vi "PID Sample Test.vi"(8 "error in":errorcluster, 11 "classes in":T3) -> (0 "error out":errorcluster, 3 "classes out":T3)   [LabVIEW 2011]
uses:
  Controls/Class Objects.ctl
  Modules/File/Configuration/Configuration.lvclass
  Modules/Hardware/Power Supply/Power Supply.lvclass
  Modules/Hardware/Mass Flow Controller/Mass Flow Controller.lvclass
  Modules/Hardware/Valve Controller/Valve Controller.lvclass
  Modules/Hardware/Multimeter/Multimeter.lvclass
  Modules/Hardware/Vapour Generator/Vapour Generator.lvclass
  Modules/File/TDMS/TDMS.lvclass
  Modules/Hardware/PID/PID.lvclass
  Modules/Hardware/Owlstone GEN-SYS/Gen-Sys Setpoints.ctl
  Modules/Hardware/Vapour Generator/Gas Output.ctl
  Modules/Hardware/Owlstone GEN-SYS/Owlstone GEN-SYS.lvclass
  Functional Global Data/Device Params Global.ctl
  Controls/TDMS File Handling.ctl
panel:
  out "Gas Output":T1 {"Relative Humidity (%)" format="%#.4g"; "Flow Rate (ml/min)" format="%#.0f"; "Concentration (ppm)" format="%#.2g"}
  in  "Owlstone-GEN-SYS Setpoints":T2={"OVG-4"={"Oven Temperature"=25, "Sample Flow Rate"=50, "Split Flow Status"=0, "Split Flow Rate"=300}, "OHG-4"={"Wet Air Flow"=300}} {"OHG-4"."Wet Air Flow" min=300 max=3000 scale=300.0..3000.0; "OVG-4"."Split Flow Status" items=["Closed", "Open"]; "OVG-4"."Split Flow Rate" min=300 max=3000 scale=300.0..3000.0; "OVG-4"."Sample Flow Rate" min=50 max=500 scale=50.0..500.0; "OVG-4"."Oven Temperature" min=25 max=100 scale=25.0..100.0}
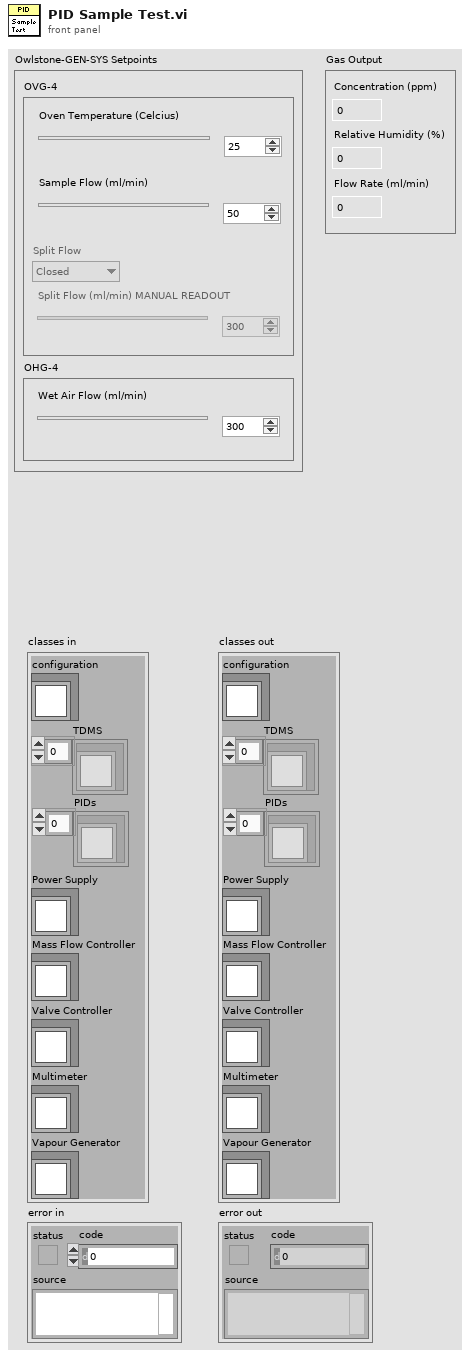
[diagram p1: front panel]
types:
  T1 = typedef "Vapour Generator.lvclass/Gas Output.ctl" = cluster{"Concentration (ppm)":dbl, "Flow Rate (ml/min)":dbl, "Relative Humidity (%)":dbl}
  T2 = typedef "Owlstone GEN-SYS.lvclass/Gen-Sys Setpoints.ctl" = cluster{"OVG-4":cluster{"Oven Temperature":i32, "Sample Flow Rate":i32, "Split Flow Status":u16, "Split Flow Rate":i32}, "OHG-4":cluster{"Wet Air Flow":i32}}
  T3 = typedef "Class Objects.ctl" = cluster{"configuration":refnum<class "Configuration.lvclass">, "TDMS":refnum<class "TDMS.lvclass">[], "Power Supply":refnum<class "Power Supply.lvclass">, "Mass Flow Controller":refnum<class "Mass Flow Controller.lvclass">, "Valve Controller":refnum<class "Valve Controller.lvclass">, "Multimeter":refnum<class "Multimeter.lvclass">, "Vapour Generator":refnum<class "Vapour Generator.lvclass">, "PIDs":refnum<class "PID.lvclass">[]}
  T4 = typedef "Device Params Global.ctl" = enum16{"Initialize", "Get Device Settings", "Get Device Connections", "Set Device Settings", "Set Device Connections", "Get All Device Properties"}
  T5 = typedef "TDMS File Handling.ctl" = enum16{"Add TDMS File", "Get Active TDMS File", "Set Active TDMS File", "Set Active TDMS File Index"}
  T6 = typedef "Device Settings.ctl" = cluster{"PID":cluster{"B-M PID":T7, "INL PID":T8}, "Power Supply":cluster{"Source Value":dbl, "Source Value Units":T9, "Source Mode":T10, "Limits":T11, "Output":bool}, "Mass Flow Controller":cluster{"MFC Flow Rate":dbl, "MFC Valve Status":T14}, "Valve Controller":cluster{"Valve Assembly":T15}, "Multimeter":cluster{"Agilent 3458A":cluster{"Measurement Configuration":T17, "Measurement Integration":T18}}, "Vapour Generator":cluster{"Owlstone Permeation Tube":T19, "Owlstone GEN-SYS Setpoints":T2}}
  T7 = typedef "Baseline Mocon piD-Tech plus.lvclass/Settings.ctl" = cluster{"Detector Sampling Frequency":dbl}
  T8 = typedef "INL PID.lvclass/Settings.ctl" = cluster{"Sampling Frequency":dbl, "Integration Time":dbl, "Integration Periods":u8, "Grid Voltage":dbl}
  T9 = typedef "Power Supply.lvclass/Source Units.ctl" = enum16{"volts", "millivolts", "microvolts", "amps", "milliamps", "microamps", "nanoamps"}
  T10 = typedef "Power Supply.lvclass/Source Mode.ctl" = enum16{"Volts", "Current"}
  T11 = typedef "Power Supply.lvclass/Protection Limits.ctl" = cluster{"Voltage Limit":dbl, "Voltage Limit Units":T12, "Current Limit":dbl, "Current Limit Units":T13, "Voltage Trip/Cmpl":dbl, "Voltage Trip/Cmpl Units":T12, "Current Trip/Cmpl":dbl, "Current Trip/Cmpl Units":T13}
  T12 = typedef "Power Supply.lvclass/Voltage Units.ctl" = enum16{"volts", "millivolts", "microvolts"}
  T13 = typedef "Power Supply.lvclass/Current Units.ctl" = enum16{"amps", "milliamps", "microamps", "nanoamps"}
  T14 = typedef "Mass Flow Controller.lvclass/Valve Status.ctl" = enum16{"Open", "Closed"}
  T15 = typedef "Valve Controller.lvclass/Valve Assembly.ctl" = cluster{"Valve 1":T16, "Valve 2":T16, "Valve 3":T16, "Valve 4":T16, "Valve 5":T16}
  T16 = typedef "Valve Controller.lvclass/Status.ctl" = u16
  T17 = typedef "Agilent 3458A.lvclass/Measurement Configuration.ctl" = cluster{"Function":enum16{"DC Voltage", "AC Voltage", "AC + DC Voltage", "DC Current", "AC Current", "AC + DC Current", "2-Wire Resistance", "4-Wire Resistance", "Frequency", "Period", "Direct Sampling DC", "Direct Sampling AC", "Sub-Sampling DC", "Sub-Sampling AC"}, " Manual Resolution":enum16{"4.5", "5.5", "6.5", "7.5", "8.5"}, "Frequency Source":enum16{"AC + DC Current", "AC + DC Voltage", "AC Current", "AC Voltage"}, "Auto Range":enum16{"OFF", "ON", "ONCE"}}
  T18 = typedef "Agilent 3458A.lvclass/Measurement Integration.ctl" = cluster{"Power Line Cycles":dbl}
  T19 = typedef "Owlstone GEN-SYS.lvclass/Permeation Tube.ctl" = cluster{"Tube":T20, "Molecular Weight":dbl, "Calibration Temperature\n(Celcius)":i32, "Permeation Rate \n(ng/min)":i32}
  T20 = typedef "Owlstone GEN-SYS.lvclass/Permeation Tube Gas.ctl" = enum16{"Isobutylene 27 Nov 2012", "Ammonia 29 Sep 2012", "DMMP Tube A 3 July 2014", "DMMP Tube B 3 July 2014"}
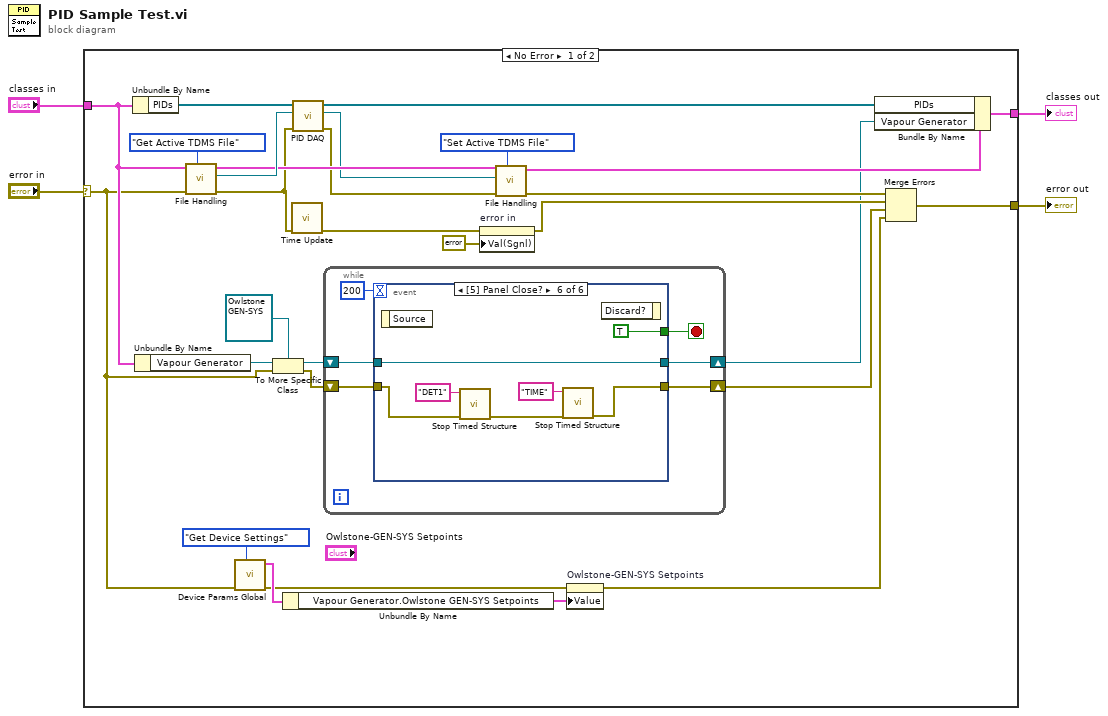
[diagram p0: block diagram]
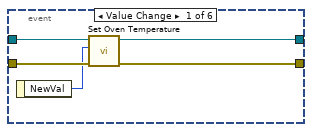
[diagram p2: hidden frame]
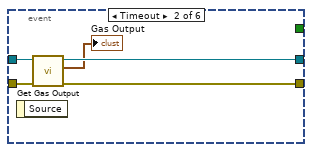
[diagram p3: hidden frame]
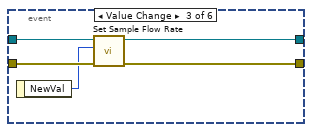
[diagram p4: hidden frame]
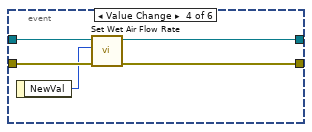
[diagram p5: hidden frame]
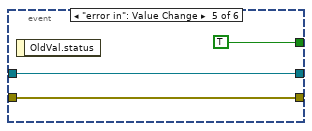
[diagram p6: hidden frame]
diagram:
  n1 = case shown="No Error" "error in" {
    selector: "error in" -> [w6 w71]
    tunnel: [w32 w71] -> w4
    tunnel: "classes in" -> [w31 w70]
    tunnel: [w33 w70] -> w1
    frame No Error {
      n2 = Unbundle By Name(w31) -> ("PIDs"=w8:refnum<class "PID.lvclass">[])
      n3 = Unbundle By Name(w31) -> ("Vapour Generator"=w12:refnum<class "Vapour Generator.lvclass">)
      n4 = call "File Handling.vi"("TDMS File Handling"=TDMS_File_Handling."Get Active TDMS File", "error in"=w6, "Class objects"=w31) -> ("error out"=w15:errorcluster, "TDMS File"=w21:refnum<class "TDMS.lvclass">, "Class objects"=w20:T3)  [unwired: 6 in]
      n5 = call "Device Params Global.vi"("action"=Device_Params_Global."Get Device Settings", "error in"=w6) -> ("error out"=w13:errorcluster, "Device Settings OUT"=w17:T6)  [unwired: 7 in, 1 out]
      n6 = To More Specific Class(target class=refnum<class "Owlstone GEN-SYS.lvclass"> refnum ("Owlstone GEN-SYS.lvclass"), reference=w12, error in=w6) -> (specific class reference=w10:refnum<class "Owlstone GEN-SYS.lvclass">, error out=w9:errorcluster)
      n7 = Unbundle By Name(w17) -> ("Vapour Generator.Owlstone GEN-SYS Setpoints"=w14:T2)
      n8 = call "Time Update.vi"("error in"=w15) -> ("error out"=w22:errorcluster)  [unwired: 10 in]
      n9 = call "PID DAQ.vi"("error in"=w15, "TDMS in"=w21, "PIDs"=w8) -> ("error out"=w16:errorcluster, "TDMS out"=w19:refnum<class "TDMS.lvclass">, "PIDs"=w7:refnum<class "PID.lvclass">[])  [unwired: 6 in]
      n10 = while {
        shift-right: [w37] -> w23
        shift-left: w10 -> [w39]
        shift-right: [w36] -> w25
        shift-left: w9 -> [w38]
        stop <- w35 stop-if-true
        n11 = event shown="[5] Panel Close?" {
          selector: _ -> [_ _ _ _ _ _]
          dyn-events: _ -> [_ _ _ _ _ _]
          timeout: 200 -> [_ _ _ _ _ _]
          tunnel: w39 -> [w40 w49 w54 w59 w60 w68]
          tunnel: w38 -> [w43 w48 w53 w58 w61 w69]
          tunnel: [w44 w47 w51 w56 w60 w68] -> w37
          tunnel: [w41 w46 w50 w55 w61 w64] -> w36
          tunnel: [_ _ _ _ TRUE TRUE] -> w35
          event Value Change {
            n12 = event-data() -> ("NewVal"=w42:i32)  [unwired: 1 in]
            n13 = call "Set Oven Temperature.vi"("error in"=w43, "Oven Temperature"=w42, "OVG In"=w40) -> ("error out"=w41:errorcluster, "OVG Out"=w44:refnum<class "Owlstone GEN-SYS.lvclass">)  [unwired: 7 in]
          }
          event Timeout {
            n14 = event-data() -> ()  [unwired: 1 in, 1 out]
            n15 = call-dynamic "Get Gas Output.vi"("error in"=w48, "Owlstone OVG-4 in"=w49) -> ("error out"=w46:errorcluster, "Output"=→"Gas Output":T1, "Owlstone OVG-4 out"=w47:refnum<class "Owlstone GEN-SYS.lvclass">)  [unwired: 7 in]
          }
          event Value Change {
            n16 = event-data() -> ("NewVal"=w52:i32)  [unwired: 1 in]
            n17 = call "Set Sample Flow Rate.vi"("error in"=w53, "Sample Flow"=w52, "OVG In"=w54) -> ("error out"=w50:errorcluster, "OVG Out"=w51:refnum<class "Owlstone GEN-SYS.lvclass">)  [unwired: 7 in]
          }
          event Value Change {
            n18 = event-data() -> ("NewVal"=w57:i32)  [unwired: 1 in]
            n19 = call "Set Wet Air Flow Rate.vi"("error in"=w58, "Wet Air Flow Rate (ml/min)"=w57, "OVG In"=w59) -> ("error out"=w55:errorcluster, "OVG Out"=w56:refnum<class "Owlstone GEN-SYS.lvclass">)  [unwired: 7 in]
          }
          event "error in": Value Change {
            n20 = event-data() -> ()  [unwired: 1 in, 1 out]
          }
          event Panel Close? {
            n21 = event-data() -> ()  [unwired: 1 in, 1 out]
            n22 = call <vilib>:"Stop Timed Structure.vi"("error in (no error)"=w69, "name"="DET1") -> ("error out"=w65:errorcluster)  [unwired: 9 in]
            n23 = call <vilib>:"Stop Timed Structure.vi"("error in (no error)"=w65, "name"="TIME") -> ("error out"=w64:errorcluster)  [unwired: 9 in]
            n24 = event-data() -> ()  [unwired: 2 in, 1 out]
          }
        }
      }
      n25 = property on="error in" class="Clust (strict)"(error in=w22, "Val(Sgnl)"=errorcluster {"status"=FALSE, "code"=0, "source"=""} ("Value (Signaling)")) -> (error out=w26:errorcluster)  [unwired: 1 in, 1 out]
      n26 = call "File Handling.vi"("TDMS File Handling"=TDMS_File_Handling."Set Active TDMS File", "error in"=w16, "TDMS File"=w19, "Class objects"=w20) -> ("error out"=w28:errorcluster, "Class objects"=w24:T3)  [unwired: 5 in, 1 out]
      n27 = property on="Owlstone-GEN-SYS Setpoints" class="Clust (strict)"(error in=w13, "Value"=w14) -> (error out=w5:errorcluster)  [unwired: 1 in, 1 out]
      n28 = Bundle By Name(cluster=w24, "PIDs"=w7, "Vapour Generator"=w23) -> (w33:T3)
      n29 = Merge Errors(w28, w26, w25, w5) -> (w32:errorcluster)
    }
    frame Error {
    }
  }
  "error out" <- w4
  "classes out" <- w1
